vi "DisplayMAXandTOF.vi"(10 "TOF":dbl[][](graph), 11 "Max Value":dbl[][](graph)) -> ()   [LabVIEW 2022 SP3]
panel:
  in  "ExitSendCmd":bool
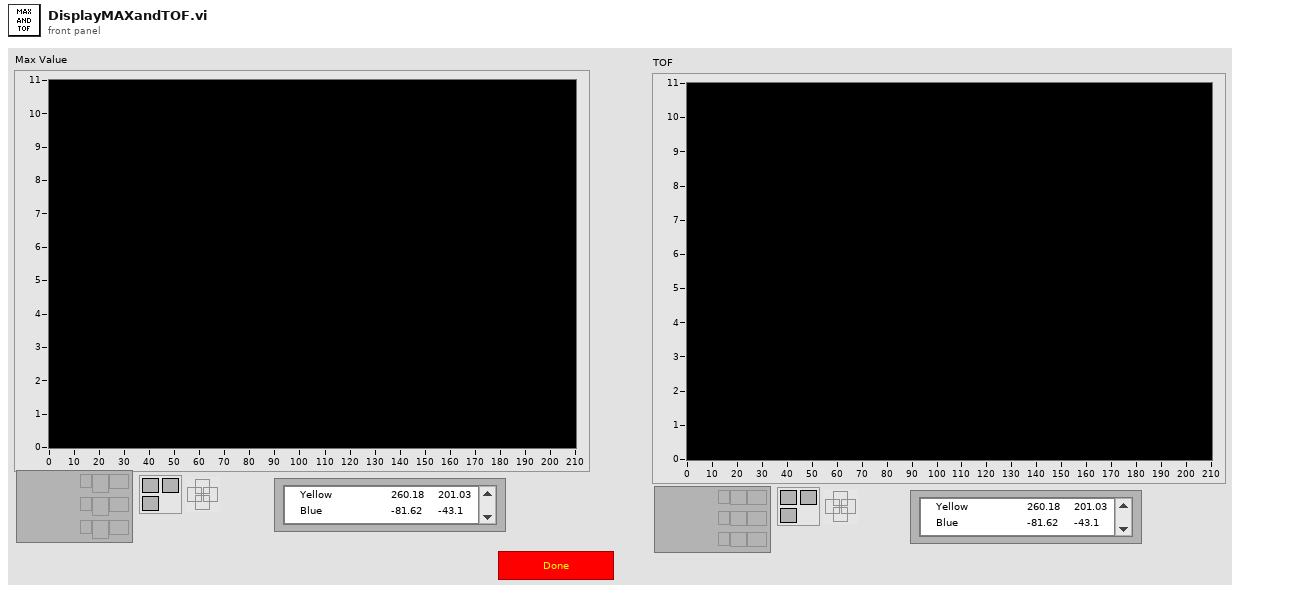
[diagram p1: front panel]
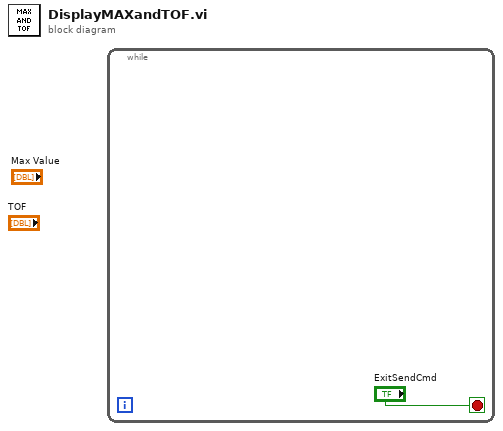
[diagram p0: block diagram]
diagram:
  n1 = while {
    stop <- "ExitSendCmd" stop-if-true
  }
